vi "signal_carre.vi"() -> ()   [LabVIEW 2010]
panel:
  in  "Numérique":dbl
  out "Numeric":i32
  out "Booléen":bool
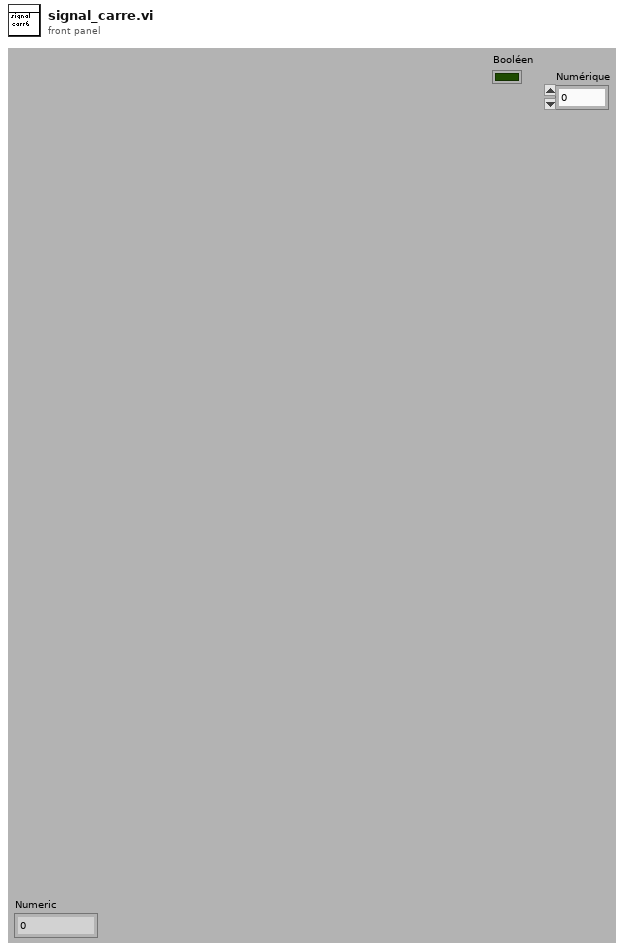
[diagram p1: front panel]
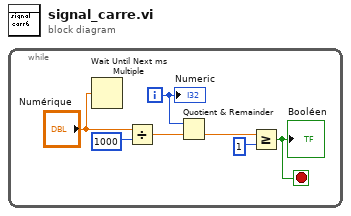
[diagram p0: block diagram]
diagram:
  n1 = while {
    i -> [w2]
    stop <- w1 stop-if-true
    n2 = Wait Until Next ms Multiple(millisecond multiple="Numérique") -> ()  [unwired: 1 out]
    n3 = Divide(x="Numérique", y=1000 ("Count(Ticks)")) -> (x/y=w6:dbl)
    n4 = Quotient & Remainder(x=w2, y=w6) -> (floor(x/y)=w3:dbl)  [unwired: 1 out]
    n5 = Greater Or Equal?(x=w3, y=1 ("Count(Ticks)")) -> (x >= y?=w1:bool)
    "Booléen" <- w1
    "Numeric" <- w2
  }
